vi "Configure Serial Bus (CAN - Trigger).vi"(0 "VISA resource name":refnum<visa-resource-name>, 1 "Data Pattern (XXXXXXXX)":string="XXXXXXXX", 2 "ID Pattern (XXXXXXXXXXX)":string="XXXXXXXXXXX", 5 "Serial Bus Name (1: Serial Bus 1)":i32(ring)=1 items=["Serial Bus 1"=1, "Serial Bus 2"=2], 7 "Trigger Condition (0: SOF)":i32(ring) items=["SOF", "Data", "Error", "ID Data", "ID Either", "ID Remote", "All Error", "Overload", "ACK Error", "Message", "Message and Signal"], 9 "Definition (0: CAN_H)":i32(ring) items=["CAN_H", "Diff High", "CAN_L", "Rx", "Tx", "Diff Low"], 11 "error in (no error)":errorcluster, 12 "Data Length (1)":i32=1, 13 "ID Mode (0: Standard)":i32(ring) items=["Standard", "Extended"]) -> (4 "VISA resource name out":refnum<visa-resource-name>, 15 "error out":errorcluster)   [LabVIEW 2023, in "Keysight-DSQx3014T.lvlib"]
doc: "Configures the trigger settings of CAN bus."
uses:
  Keysight-DSQx3014T.lvlib
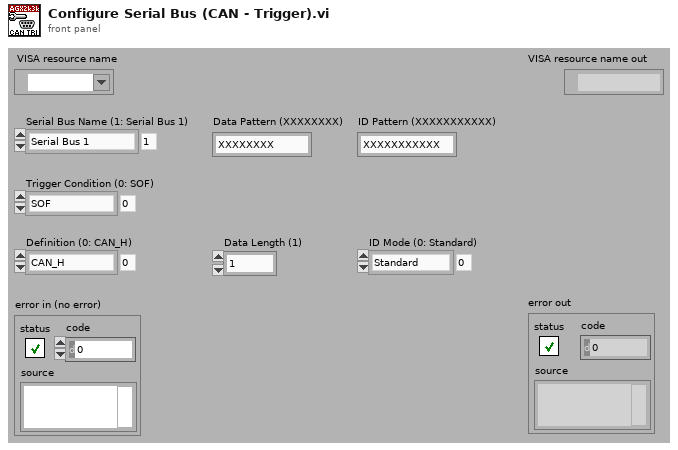
[diagram p1: front panel]
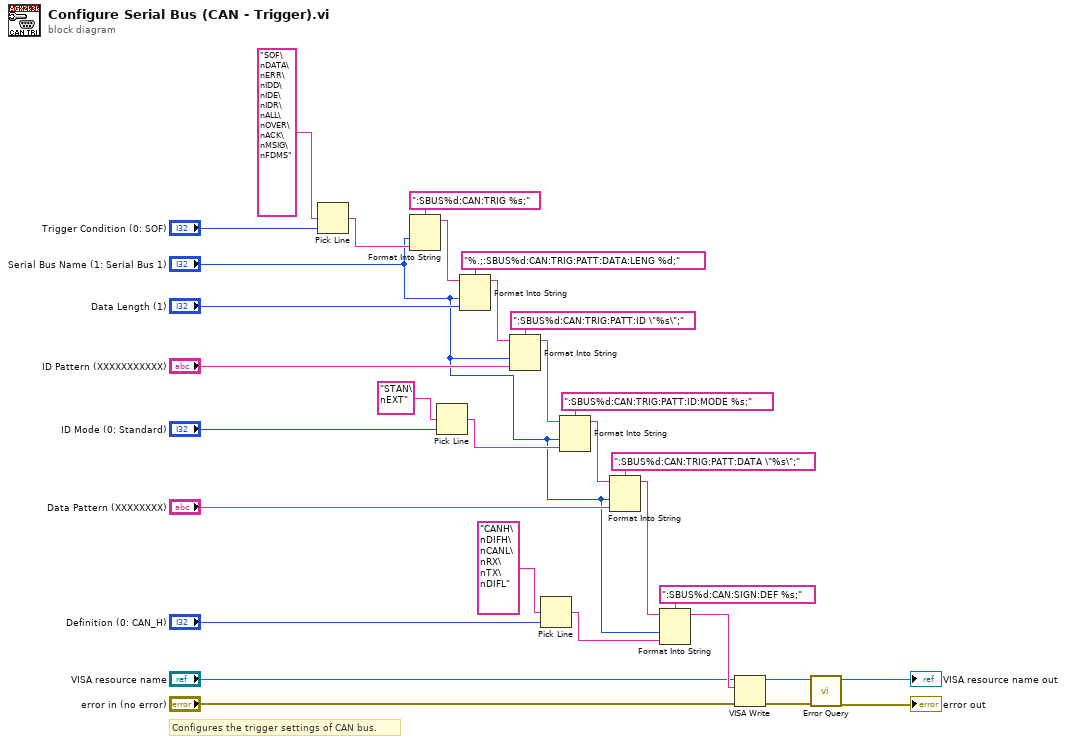
[diagram p0: block diagram]
diagram:
  # "Configures the trigger settings of CAN bus."
  n1 = Pick Line(multi-line string="SOF\nDATA\nERR\nIDD\nIDE\nIDR\nALL\nOVER\nACK\nMSIG\nFDMS", line index="Trigger Condition (0: SOF)") -> (output string=w28:string)  [unwired: 1 out]
  n2 = Format Into String(format string=":SBUS%d:CAN:TRIG %s;", "Serial Bus Name (1: Serial Bus 1)", w28) -> (resulting string=w27:string)  [unwired: 2 in, 1 out]
  n3 = Pick Line(multi-line string="STAN\nEXT", line index="ID Mode (0: Standard)") -> (output string=w17:string)  [unwired: 1 out]
  n4 = Format Into String(format string="%.;:SBUS%d:CAN:TRIG:PATT:DATA:LENG %d;", initial string=w27, "Serial Bus Name (1: Serial Bus 1)", "Data Length (1)") -> (resulting string=w24:string)  [unwired: 1 in, 1 out]
  n5 = Format Into String(format string=":SBUS%d:CAN:TRIG:PATT:ID \"%s\";", initial string=w24, "Serial Bus Name (1: Serial Bus 1)", "ID Pattern (XXXXXXXXXXX)") -> (resulting string=w19:string)  [unwired: 1 in, 1 out]
  n6 = Pick Line(multi-line string="CANH\nDIFH\nCANL\nRX\nTX\nDIFL", line index="Definition (0: CAN_H)") -> (output string=w9:string)  [unwired: 1 out]
  n7 = Format Into String(format string=":SBUS%d:CAN:TRIG:PATT:ID:MODE %s;", initial string=w19, "Serial Bus Name (1: Serial Bus 1)", w17) -> (resulting string=w16:string)  [unwired: 1 in, 1 out]
  n8 = Format Into String(format string=":SBUS%d:CAN:TRIG:PATT:DATA \"%s\";", initial string=w16, "Serial Bus Name (1: Serial Bus 1)", "Data Pattern (XXXXXXXX)") -> (resulting string=w11:string)  [unwired: 1 in, 1 out]
  n9 = Format Into String(format string=":SBUS%d:CAN:SIGN:DEF %s;", initial string=w11, "Serial Bus Name (1: Serial Bus 1)", w9) -> (resulting string=w8:string)  [unwired: 1 in, 1 out]
  n10 = VISA Write(VISA resource name="VISA resource name", write buffer=w8, error in (no error)="error in (no error)") -> (VISA resource name out=w5:refnum<visa-resource-name>, error out=w4:errorcluster)  [unwired: 1 out]
  n11 = call "Error Query.vi"("error in (no error)"=w4, "VISA resource name"=w5) -> ("error out"=→"error out":errorcluster, "VISA resource name out"=→"VISA resource name out":refnum<visa-resource-name>)  [unwired: 8 out]
